vi "GetActiveFieldName.vi"(1 "protobuf index":i32) -> (0 "oneof field name":string)   [LabVIEW 2019, in "grpc-xnet_client.lvlib" / "nixnet_grpc_FrameBufferResponse_frame.lvclass"]
uses:
  nixnet_grpc_FrameBufferResponse_frame.lvclass
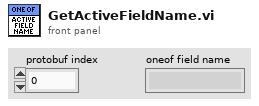
[diagram p1: front panel]
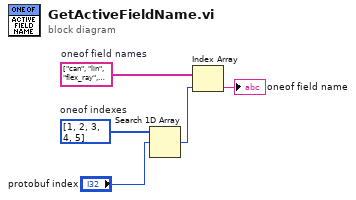
[diagram p0: block diagram]
diagram:
  w5 = string[] ["can", "lin", "flex_ray", "j1939", "enet"]  # oneof field names
  w4 = i32[] [1, 2, 3, 4, 5]  # oneof indexes
  n1 = Search 1D Array(1D array=w4, element="protobuf index") -> (index of element=w2:i32)  [unwired: 1 in]
  n2 = Index Array(array=w5, index=w2) -> (element=→"oneof field name":string)
